vi "setSampling.vi"(8 "error in (no error)":errorcluster, 10 "sampling":T1={"Fs"=204789.0, "#s"=15753}, 11 "Instrument.LockinAPI in":refnum<class "Instrument.LockinAPI.lvclass">) -> (0 "error out":errorcluster, 3 "Instrument.LockinAPI out":refnum<class "Instrument.LockinAPI.lvclass">)   [LabVIEW 2019, in "Instrument.LockinAPI.lvclass"]
doc: "API to put lockin into remote mode.\n\nIf address=\"\", this API reads from localhost\nIf address is remote lockin, you need to add this computer to allowed whitelist on the lockin computer you are trying to access."
uses:
  Instrument.LockinAPI.lvclass
  Typedefs/LockinAPI.Sampling.Sampling--Cluster.ctl
  C:/Users/patrick/Documents/GitHub/Instrument-Framework/lvsrc/Instrument/Instrument.lvclass
  Typedefs/LockinAPI.Commands--Enum.ctl
  Typedefs/LockinAPI.Sampling.FsMode--enum.ctl
  06eb4e12-939d-46df-a9b7-83f1e1fdd163.vi
  06eb4e12-939d-46df-a9b7-83f1e1fdd163.vi/c1229636-4044-4d8b-ac1e-2d6b8056063d.vi
  06eb4e12-939d-46df-a9b7-83f1e1fdd163.vi/c1229636-4044-4d8b-ac1e-2d6b8056063d.vi/34dbae93-0fe6-4b7d-95aa-cd44e79ba5ec.vi
  06eb4e12-939d-46df-a9b7-83f1e1fdd163.vi/c1229636-4044-4d8b-ac1e-2d6b8056063d.vi/7b3d37c5-9cf8-416c-a5da-10c254e38ae6.vi
  Instrument/Protected/Validate API method.vi
  Instrument/Private/Get RC Connection Status.vi
  Instrument/API/Send and Receive.vi
  <vilib>/Utility/Data Type/Get Type Information.vi
  <vilib>/JDP Science/JSONtext/JSON text to Variant.vi
  <vilib>/JDP Science/JSONtext/LVClass Serializer/JSONtext LVClass Serializer.lvclass
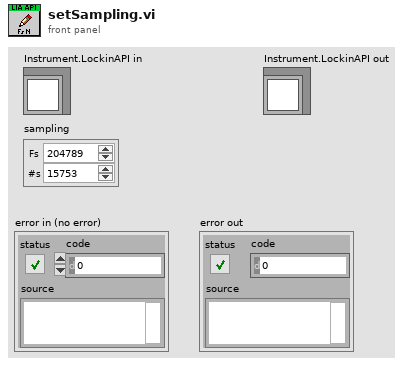
[diagram p1: front panel]
types:
  T1 = typedef "Instrument.LockinAPI.lvclass/LockinAPI.Sampling.Sampling--Cluster.ctl" = cluster{"Fs":dbl, "#s":i32}
  T2 = typedef "Instrument.LockinAPI.lvclass/LockinAPI.Sampling.FsMode--enum.ctl" = enum16{"Manual", "Auto Fs", "Max Fs"}
  T3 = typedef "Instrument.LockinAPI.lvclass/LockinAPI.Commands--Enum.ctl" = enum16{"setAI", "setAO", "setAO_Amplitude", "setAO_DC", "setAO_Frequency", "setAO_Phase", "setAO_Function", "setAO_I+", "setREF", "setREF_Frequency", "setREF_Phase", "setREF_TC", "setREF_Roll-Off", "setDAQ", "setSampling", "setOffset", "setState", "getState", "getAO", "getAI", "getResults", "getSampling", "getAOconfig", "getREFconfig", "setInputGain", "setOutputGain", "getInputGain", "getOutputGain", "setSamplingMode", "getSamplingMode", "setSweep", "setSweepTime", "setSweepTable", "getStatus", "getSweepResults", "getSweepWaveforms", "startSweep", "stopSweep", "setAUX", "getAUX"}
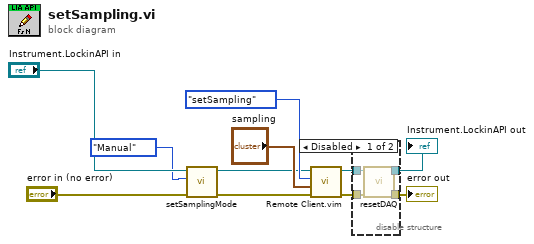
[diagram p0: block diagram]
diagram:
  n1 = call-dynamic "setSamplingMode.vi"("error in (no error)"="error in (no error)", "Fs Mode"=LockinAPI.Sampling.FsMode--enum."Manual", "Instrument.LockinAPI in"="Instrument.LockinAPI in") -> ("error out"=w7:errorcluster, "Instrument.LockinAPI out"=w6:refnum<class "Instrument.LockinAPI.lvclass">)  [unwired: 7 in]
  n2 = call "Remote Client.vim"("error in (no error)"=w7, "Data in"="sampling", "Command in"=LockinAPI.Commands--Enum."setSampling" ("Command"), "Instrument in"=w6) -> ("error out"=w2:errorcluster, "Instrument out"=w5:refnum<class "Instrument.LockinAPI.lvclass">)  [unwired: 4 in, 2 out]
  n3 = disable-structure shown="Disabled" {
    disable-tunnel: w5 -> [w15 w17]
    disable-tunnel: [w14 w17] -> w4
    disable-tunnel: [w13 w16] -> w3
    disable-tunnel: w2 -> [w12 w16]
    frame Disabled {
      n4 = call-dynamic "resetDAQ.vi"("error in (no error)"=w12, "Instrument.LockinAPI in"=w15) -> ("error out"=w13:errorcluster, "Instrument.LockinAPI out"=w14:refnum<class "Instrument.LockinAPI.lvclass">)  [unwired: 8 in]
    }
    frame Enabled {
    }
  }
  "error out" <- w3
  "Instrument.LockinAPI out" <- w4
